vi "Python@GetPoint__Parameter.vi"(1 "ParamterIn":string) -> (0 "ParamterOut":string)   [LabVIEW 2020]
panel:
  in  "ARCOSName":string(combo) caption="ARCOSName="
  in  "PythonVariable":string(combo)
  in  "Confirm":bool
  # "Python@GetPoint $PythonPoint(,ARCOSName=)"
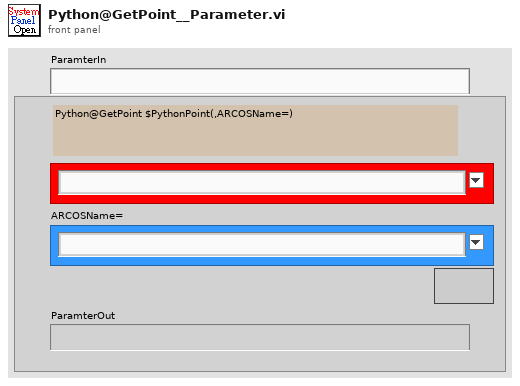
[diagram p1: front panel]
types:
  T1 = enum16{"Get", "UpdatePointS", "Init", "UpdateIndex", "GetCurrent&Index+1", "GetWithIndex", "ChkLast", "GetCurrent"}
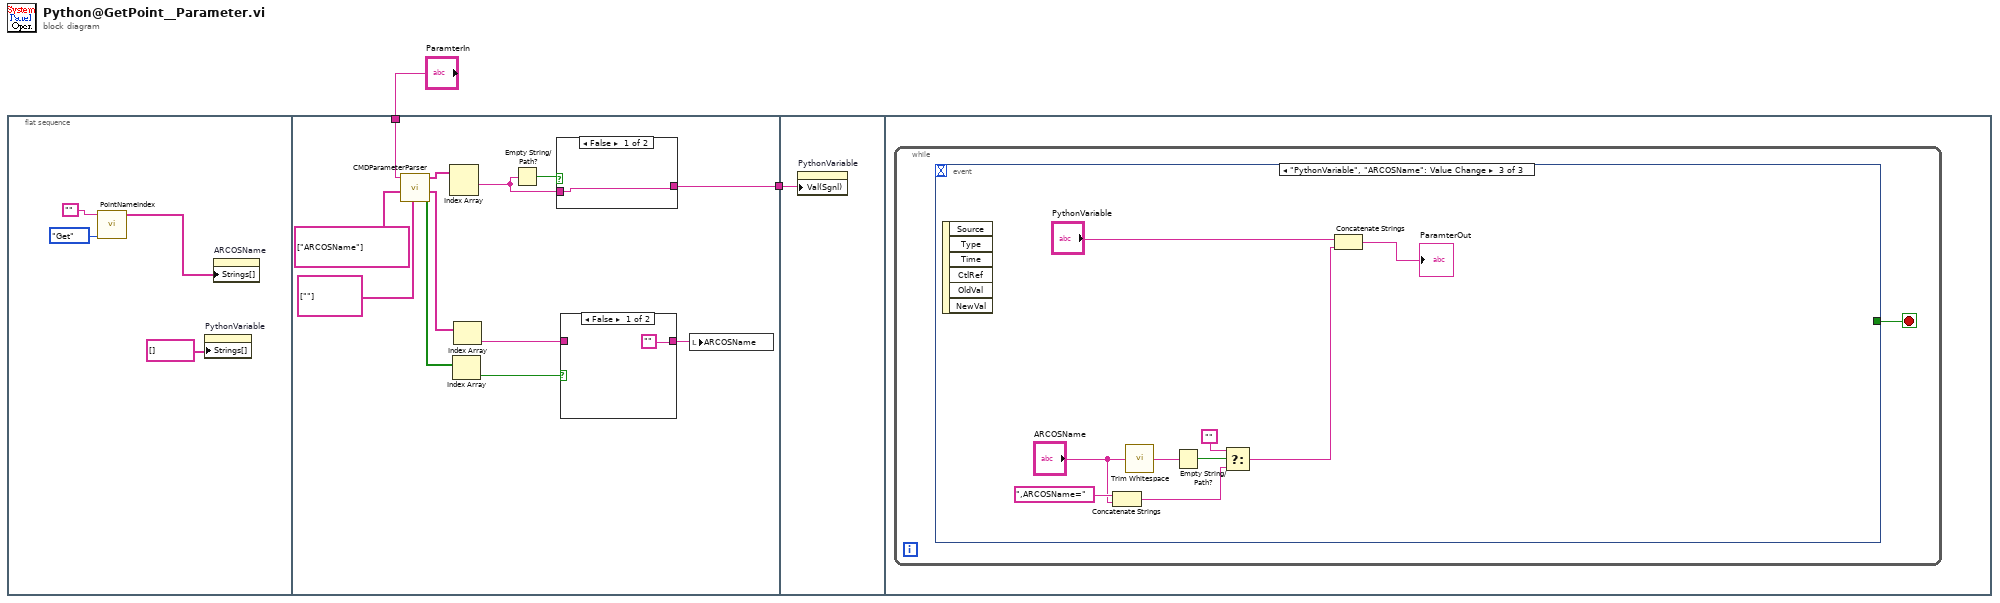
[diagram p0: block diagram]
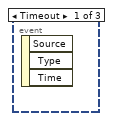
[diagram p4: hidden frame]
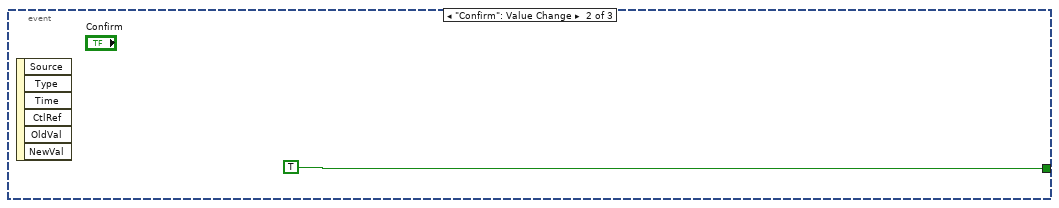
[diagram p5: hidden frame]
diagram:
  n1 = flat-sequence {
    tunnel: "ParamterIn" -> [w15]
    tunnel: [w17] -> w1
    tunnel: w1 -> [w23]
    frame #0 {
      n2 = call "PointNameIndex.vi"("OP"=T1."Get", "PointName"="") -> ("PointNameList"=w3:string[])  [unwired: 4 in, 5 out]
      n3 = property on="PythonVariable" class="CmbBox"("Strings[]"=string[] [] ("Strings []")) -> ()  [unwired: 2 in, 2 out]
      n4 = property on="ARCOSName" class="CmbBox"("Strings[]"=w3) -> ()  [unwired: 2 in, 2 out]
    }
    frame #1 {
      n5 = call "CMDParameterParser.vi"("DeafultValues"=string[] [""], "RequiredKeys"=string[] ["ARCOSName"], "CMDParameter"=w15) -> ("KeyFind?"=w10:bool[], "KeyValues"=w11:string[], "Input"=w14:string[])  [unwired: 6 in]
      n6 = Index Array(array=w14) -> (element #1=w16:string)  [unwired: 2 in, 1 out]
      n7 = Index Array(array=w10) -> (element=w9:bool)  [unwired: 1 in]
      n8 = Index Array(array=w11) -> (element=w8:string)  [unwired: 1 in]
      n9 = Empty String/Path?(string/path=w16) -> (empty?=w18:bool)
      n10 = case shown="False" w18 {
        tunnel: w16 -> [w21 w22]
        tunnel: [w21 w22] -> w17
        frame False {
        }
        frame True {
        }
      }
      n11 = case shown="False" w9 {
        tunnel: w8 -> [_ w20]
        tunnel: ["" w20] -> w7
        frame False {
        }
        frame True {
        }
      }
      n12 = local write "ARCOSName"(w7) -> ()
    }
    frame #2 {
      n13 = property on="PythonVariable" class="CmbBox"("Val(Sgnl)"=w23) -> ()  [unwired: 2 in, 2 out]
    }
    frame #3 {
      n14 = while {
        stop <- w24 stop-if-true
        n15 = event shown="[2] \"PythonVariable\", \"ARCOSName\": Value Change" {
          selector: _ -> [_ _ _]
          dyn-events: _ -> [_ _ _]
          timeout: _ -> [_ _ _]
          tunnel: [_ TRUE _] -> w24
          event Timeout {
            n16 = event-data() -> ()  [unwired: 1 in, 3 out]
          }
          event "Confirm": Value Change {
            n17 = event-data() -> ()  [unwired: 1 in, 6 out]
          }
          event "PythonVariable", "ARCOSName": Value Change {
            n18 = event-data() -> ()  [unwired: 1 in, 6 out]
            n19 = Concatenate Strings(",ARCOSName=" ("string"), "ARCOSName") -> (w27:string)
            n20 = call <vilib>:"Trim Whitespace.vi"("string"="ARCOSName") -> ("trimmed string"=w30:string)  [unwired: 1 in]
            n21 = Empty String/Path?(string/path=w30) -> (empty?=w29:bool)
            n22 = Select(t="", s=w29, f=w27) -> (s? t:f=w26:string)
            n23 = Concatenate Strings("PythonVariable", w26) -> (→"ParamterOut":string)
          }
        }
      }
    }
  }
